vi "Port Index Search.vi"(8 "error in":errorcluster) -> (0 "error out":errorcluster, 1 "Decimal Port Index":i32, 2 "Port Index":string, 3 "Device Description":string)   [LabVIEW 2019, in "Relay-Box.lvclass"]
uses:
  <userlib>/LevyLab/Relay Box/Relay-Box.lvclass
  <userlib>/LevyLab/Relay Box/D2XX_Functions/D2XX_Functions.lvlib
panel:
  out "Device Descriptions []":string[](array[string])
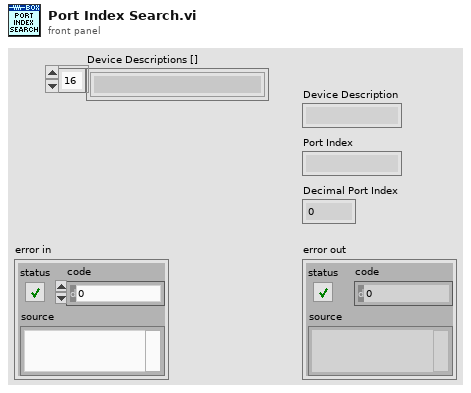
[diagram p1: front panel]
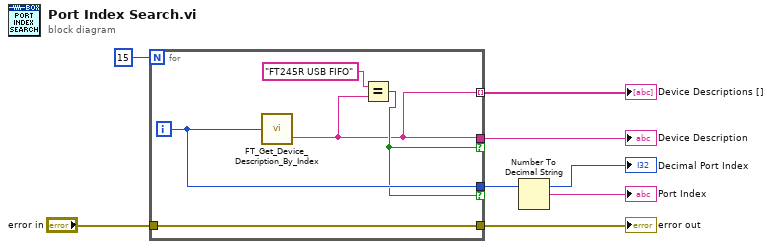
[diagram p0: block diagram]
diagram:
  n1 = for {
    N: 15 -> [_]
    tunnel: [w9] -> w6 if=w10
    tunnel: [w11] -> w2 if=w10
    tunnel: "error in" -> [w8]
    tunnel: [w8] -> w5
    tunnel: [w9] -> w3 mode=indexing
    i -> [w11]
    n2 = call <userlib>:"FT_Get_Device_Description_By_Index.vi"("Device Index"=w11) -> ("Device Description"=w9:string)  [unwired: 1 out]
    n3 = Equal?(x="FT245R USB FIFO", y=w9) -> (x = y?=w10:bool)
  }
  "Device Description" <- w6
  "error out" <- w5
  "Device Descriptions []" <- w3
  "Decimal Port Index" <- w2
  n4 = Number To Decimal String(number=w2) -> (decimal integer string=→"Port Index":string)  [unwired: 1 in]
